vi "TCP.IP Server for Ripple Detection - Experiment 5.vi"() -> ()   [LabVIEW 2021]
doc: "Demonstrates how to set up a basic TCP connection, send data to the specified port once a connection has been established, and terminate the connection once the data has been sent. This VI is designed to stop if the TCP connection is terminated. The data sent in this example is an array of random numbers."
panel:
  in  "Number of row to read \nat a time":i32=10000
  in  "File Path":path
  out "Iteration terminal":i32
  in  "Stop 2":bool
  in  "Client Closed":string="The client VI closed the connection."
  in  "Stop":bool
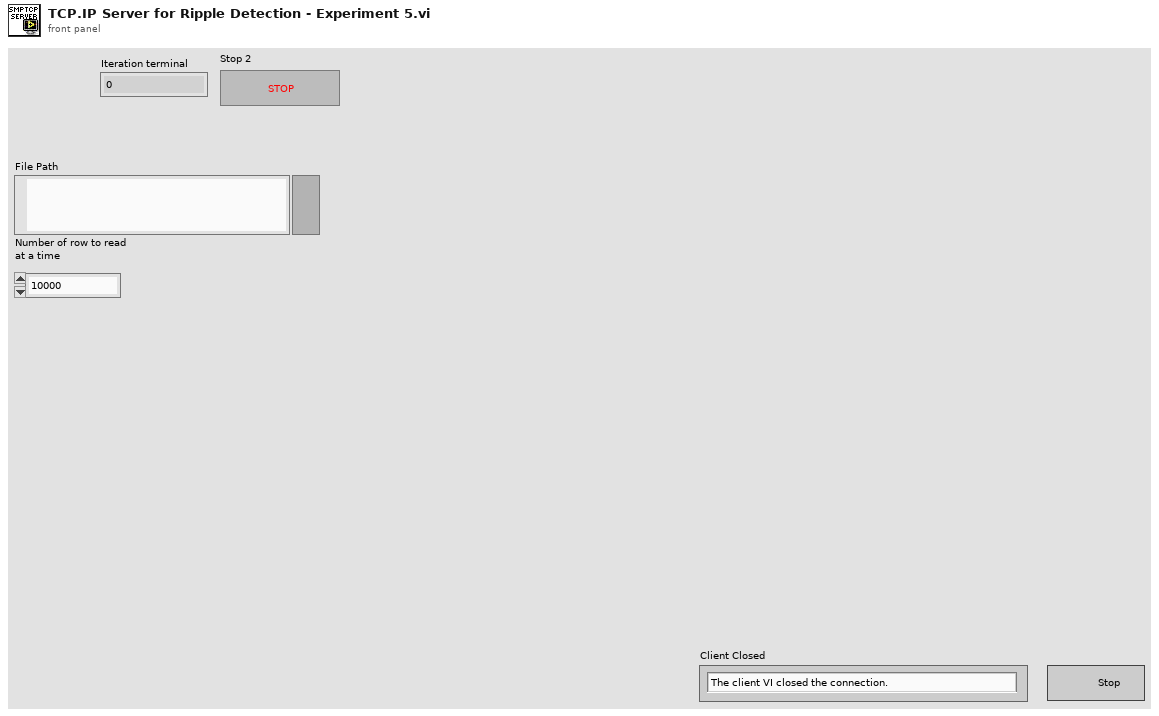
[diagram p1: front panel]
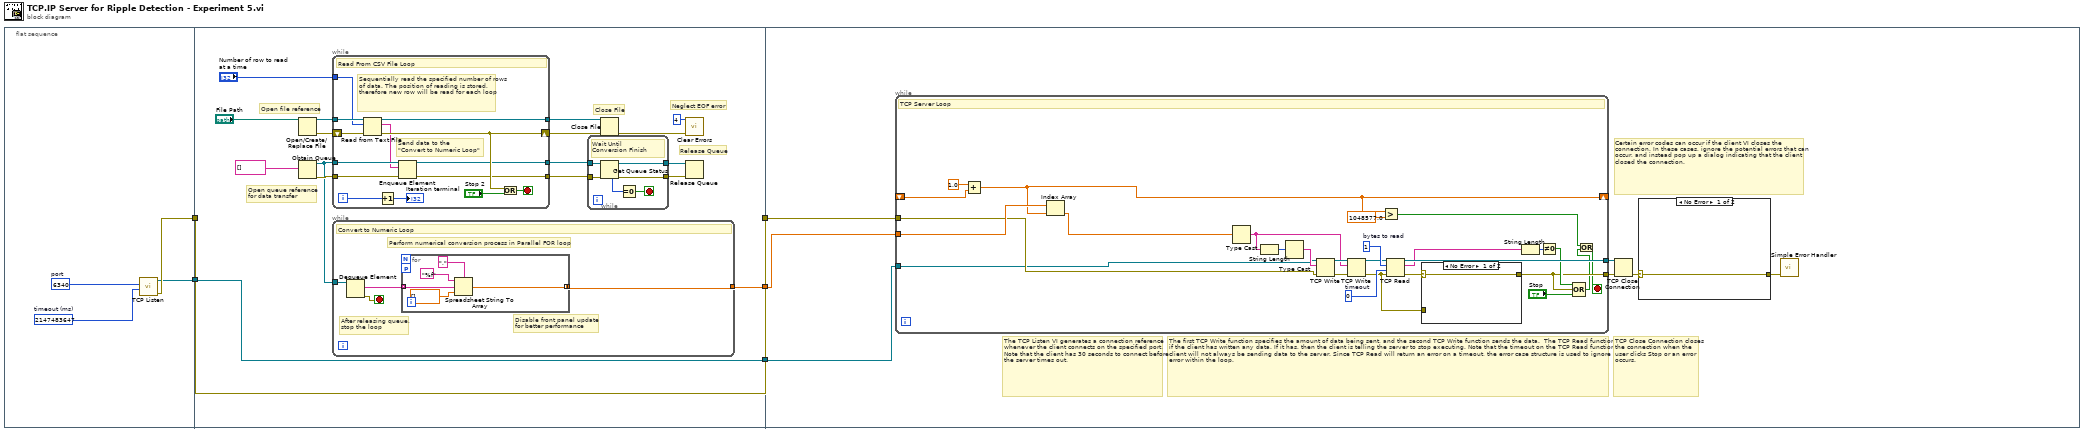
[diagram p0: block diagram]
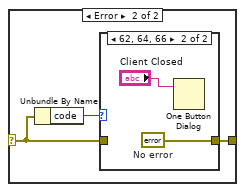
[diagram p2: hidden frame]
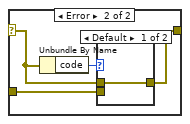
[diagram p4: hidden frame]
diagram:
  n1 = flat-sequence {
    tunnel: [w7] -> w3
    tunnel: [w6] -> w1
    tunnel: [w12] -> w5
    tunnel: [w11] -> w4
    tunnel: w3 -> [w11]
    tunnel: [w10] -> w2
    tunnel: w1 -> [w10]
    tunnel: w5 -> [w59]
    tunnel: w4 -> [w58]
    tunnel: w2 -> [w57]
    frame #0 {
      w8 = u16 6340  # port
      w9 = 2147483647  # timeout (ms)
      n2 = call <vilib>:"TCP Listen.vi"("timeout ms (wait forever: -1)"=w9, "port"=w8) -> ("error out"=w7:errorcluster, "connection ID"=w6:refnum<k5>)  [unwired: 5 in, 3 out]
    }
    frame #1 {
      # "Neglect EOF error"
      # "Release Queue"
      # "Close File"
      # "Open queue reference\nfor data transfer"
      # "Open file reference"
      n3 = Open/Create/Replace File(file path (use dialog)="File Path") -> (refnum out=w25:refnum<file>, error out=w24:errorcluster)  [unwired: 5 in, 1 out]
      n4 = Obtain Queue(element data type=string[] [] ("形式文字列")) -> (queue out=w17:refnum<queue>, error out=w18:errorcluster)  [unwired: 4 in, 1 out]
      n5 = while {
        tunnel: w25 -> [w47]
        tunnel: [w45] -> w22
        shift-right: [w40] -> w21
        shift-left: w24 -> [w46]
        tunnel: "Number of row to read \nat a time" -> [w41]
        tunnel: w17 -> [w39]
        tunnel: w18 -> [w38]
        tunnel: [w36] -> w16
        tunnel: [w35] -> w15
        i -> [w43]
        stop <- w44 stop-if-true
        # "Send data to the \n\"Convert to Numeric Loop\""
        # "Sequentially read the specified number of rows of data. The position of reading is stored, therefore new row will be read for each loop"
        # "Read From CSV File Loop"
        n6 = Read from Text File(file (use dialog)=w47, count=w41, error in=w46) -> (refnum out=w45:refnum<file>, text=w37:string[], error out=w40:errorcluster)  [unwired: 1 in, 1 out]
        n7 = Increment(x=w43) -> (x+1=→"Iteration terminal":i32)
        n8 = Enqueue Element(queue=w39, element=w37, error in (no error)=w38) -> (queue out=w36:refnum<queue>, error out=w35:errorcluster)  [unwired: 1 in, 1 out]
        n9 = Or(x=w40, y="Stop 2") -> (x .or. y?=w44:bool)
      }
      n10 = while {
        tunnel: w17 -> [w51]
        tunnel: [w48] -> w12
        stop <- w49 stop-if-true
        # "Disable front panel update \nfor better performance"
        # "After releasing queue,\nstop the loop"
        # "Perform numerical conversion process in Parallel FOR loop"
        # "Convert to Numeric Loop"
        n11 = Dequeue Element(queue=w51) -> (element=w50:string[], error out=w49:errorcluster)  [unwired: 2 in, 2 out]
        n12 = for "Forループ" {
          tunnel: w50 -> [w54] mode=indexing
          tunnel: [w52] -> w48 mode=concatenating
          workers-P: _ -> [_]
          n13 = Spreadsheet String To Array(delimiter (Tab)="," ("デリミタ（タブ）"), format string="%f" ("形式文字列"), spreadsheet string=w54, array type (2D Dbl)=dbl[] []) -> (array=w52:dbl[])
        }
      }
      n14 = while {
        tunnel: w16 -> [w33]
        tunnel: w15 -> [w32]
        tunnel: [w29] -> w13
        tunnel: [w28] -> w14
        stop <- w30 stop-if-true
        # "Wait Until \nConversion Finish"
        n15 = Get Queue Status(queue=w33, error in (no error)=w32) -> (queue out=w29:refnum<queue>, error out=w28:errorcluster, # elements in queue=w31:i32)  [unwired: 1 in, 5 out]
        n16 = Equal To 0?(x=w31) -> (x = 0?=w30:bool)
      }
      n17 = Close File(refnum=w22, error in=w21) -> (error out=w20:errorcluster)  [unwired: 1 out]
      n18 = call <vilib>:"Clear Errors.vi"("error in (no error)"=w20, "specific error code to clear (0: all)"=4) -> ()  [unwired: 4 in, 2 out]
      n19 = Release Queue(queue=w13, error in (no error)=w14) -> ()  [unwired: 1 in, 3 out]
    }
    frame #2 {
      # "TCP Close Connection closes the connection when the user clicks Stop or an error occurs."
      # "The TCP Listen VI generates a connection reference whenever the client connects on the specified port. Note that the client has 30 seconds to connect before the server times out."
      # "Certain error codes can occur if the client VI closes the connection. In these cases, ignore the potential errors that can occur, and instead pop up a dialog indicating that the client closed the connection."
      # "The first TCP Write function specifies the amount of data being sent, and the second TCP Write function sends the data.  The TCP Read function checks to see if the client has written any data. If it has, then the client is telling the server to stop executing. Note that the timeout on the TCP Read function is '0', as the client will not always be sending data to the server. Since TCP Read will return an error on a timeout, the error case structure is used to ignore the timeout error within the loop."
      n20 = while {
        tunnel: [w83] -> w61
        tunnel: [w89] -> w60
        tunnel: w59 -> [w81]
        shift-right: [w75] -> _
        shift-left: _ -> [w79]
        tunnel: w58 -> [w77]
        tunnel: w57 -> [w76]
        stop <- w71 stop-if-true
        w88 = 0  # timeout
        w91 = 1  # bytes to read
        # "TCP Server Loop"
        n21 = Add(x=1.0, y=w79) -> (x+y=w75:dbl)
        n22 = Index Array(array=w81, index=w75) -> (element=w78:dbl)
        n23 = Type Cast(x=w78) -> (*(type *) &x=w93:string)  [unwired: 1 out]
        n24 = String Length(string=w93) -> (length=w95:i32)
        n25 = Type Cast(x=w95) -> (*(type *) &x=w94:string)  [unwired: 1 out]
        n26 = TCP Write(connection ID=w76, data in=w94, error in (no error)=w77) -> (connection ID out=w97:refnum<k5>, error out=w96:errorcluster)  [unwired: 2 out]
        n27 = TCP Write(connection ID=w97, data in=w93, error in (no error)=w96) -> (connection ID out=w90:refnum<k5>, error out=w82:errorcluster)  [unwired: 2 out]
        n28 = Greater?(x=w75, y=1048577.0) -> (0:w73:bool)
        n29 = TCP Read(connection ID=w90, bytes to read=w91, error in (no error)=w82, 9:w88) -> (connection ID out=w89:refnum<k5>, data out=w86:string, error out=w84:errorcluster)  [unwired: 1 out]
        n30 = case shown="No Error" w84 {
          selector: w84 -> [w98 w101]
          tunnel: [w98 w99] -> w83
          tunnel: w82 -> [_ w100]
          frame No Error {
          }
          frame Error {
            n31 = Unbundle By Name(w101) -> ("code"=w102:i32)
            n32 = case shown="Default" w102 {
              tunnel: w101 -> [w103 _]
              tunnel: w100 -> [_ w104]
              tunnel: [w103 w104] -> w99
              frame Default {
              }
              frame 56 {
              }
            }
          }
        }
        n33 = String Length(string=w86) -> (length=w87:i32)
        n34 = Not Equal To 0?(x=w87) -> (x != 0?=w85:bool)
        n35 = Compound Arithmetic op=OR(w85, w83, "Stop") -> (w72:bool)
        n36 = Or(x=w73, y=w72) -> (x .or. y?=w71:bool)
      }
      n37 = TCP Close Connection(connection ID=w60, error in (no error)=w61) -> (error out=w62:errorcluster)  [unwired: 2 out]
      n38 = case shown="No Error" w62 {
        selector: w62 -> [w64 w66]
        tunnel: [w64 w65] -> w63
        frame No Error {
        }
        frame Error {
          n39 = Unbundle By Name(w66) -> ("code"=w67:i32)
          n40 = case shown="62, 64, 66" w67 {
            tunnel: w66 -> [w68 _]
            tunnel: [w68 w70] -> w65
            frame Default {
            }
            frame 62, 64, 66 {
              w70 = errorcluster {"status"=FALSE, "code"=0, "source"=""}  # No error
              n41 = One Button Dialog(message="Client Closed") -> ()  [unwired: 1 in, 1 out]
            }
          }
        }
      }
      n42 = call <vilib>:"Simple Error Handler.vi"("error in (no error)"=w63) -> ()  [unwired: 1 in, 8 out]
    }
  }
